vi "forLoopSample.vi"() -> ()   [LabVIEW 2025]
panel:
  out "Array 4":dbl[](array[numeric])
  in  "count 2":dbl
  out "Numeric":dbl
  out "Numeric 2":dbl
  in  "Array 3":dbl[](array[numeric])
  in  "count":dbl
  in  "Celcius":dbl(slide) scale=0.0..50.0
  out "Fahrenheit":dbl(slide) scale=0.0..120.0
  in  "check":bool
  out "iteration":dbl
  out "Waveform Chart":dbl(graph)
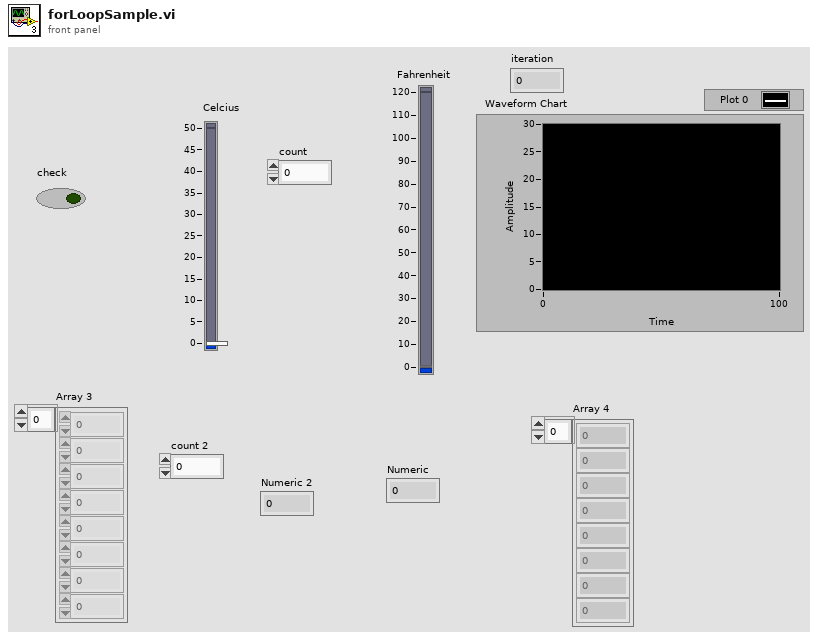
[diagram p1: front panel]
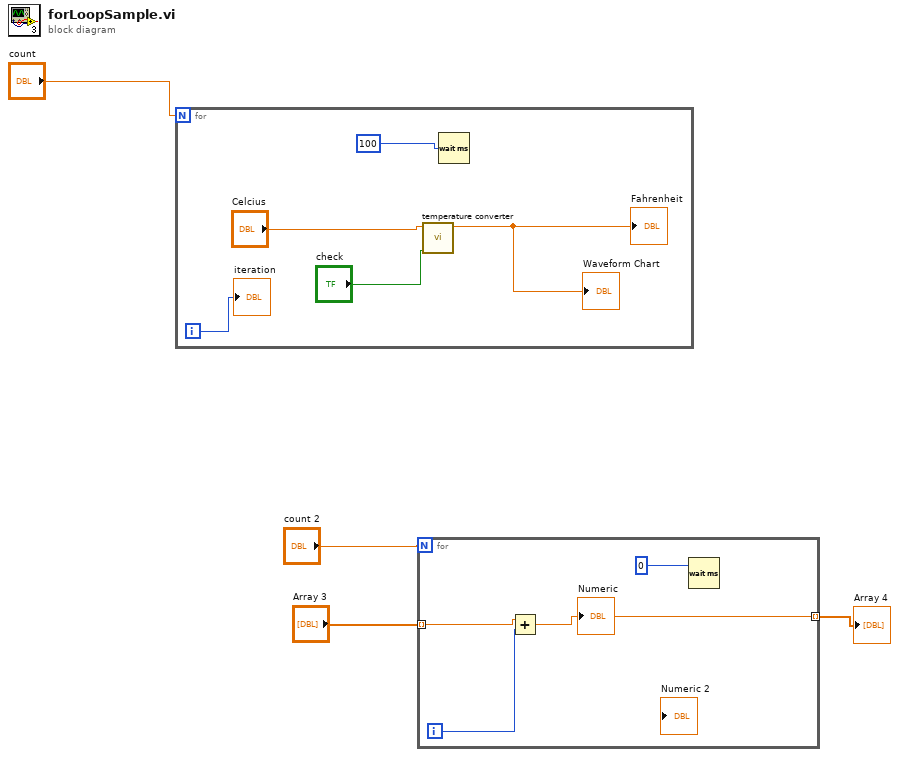
[diagram p0: block diagram]
diagram:
  n1 = for {
    N: "count" -> [_]
    i -> [w6]
    n2 = call "temperature converter.vi"("Boolean"="check", "Celcius"="Celcius") -> ("Numeric"=→"Fahrenheit" →"Waveform Chart":dbl)  [unwired: 9 in]
    n3 = Wait (ms)(milliseconds to wait=100) -> ()  [unwired: 1 out]
    "iteration" <- w6
  }
  n4 = for {
    N: "count 2" -> [_]
    tunnel: "Array 3" -> [w13] mode=indexing
    tunnel: [w11] -> w1 mode=indexing
    i -> [w12]
    n5 = Add(x=w13, y=w12) -> (x+y=w11:dbl)
    "Numeric" <- w11
    n6 = Wait (ms)(milliseconds to wait=0) -> ()  [unwired: 1 out]
  }
  "Array 4" <- w1
